vi "[Comment] Write.vi"(8 "error in (no error)":errorcluster, 11 "Graph Comment Config":T2[](array[typedef])) -> (0 "error out":errorcluster)   [LabVIEW 2019, in "Graph Tools.lvlib"]
uses:
  Graph Tools.lvlib
  [Comment] Config.ctl
  Selection VIs/controls/MarkerOptions.ctl
  <vilib>/Utility/miscctls.llb/LVPoint32TypeDef.ctl
  Selection VIs/controls/MarkerInfo.ctl
  Selection VIs/controls/markerType.ctl
panel:
  out "Coords":T1
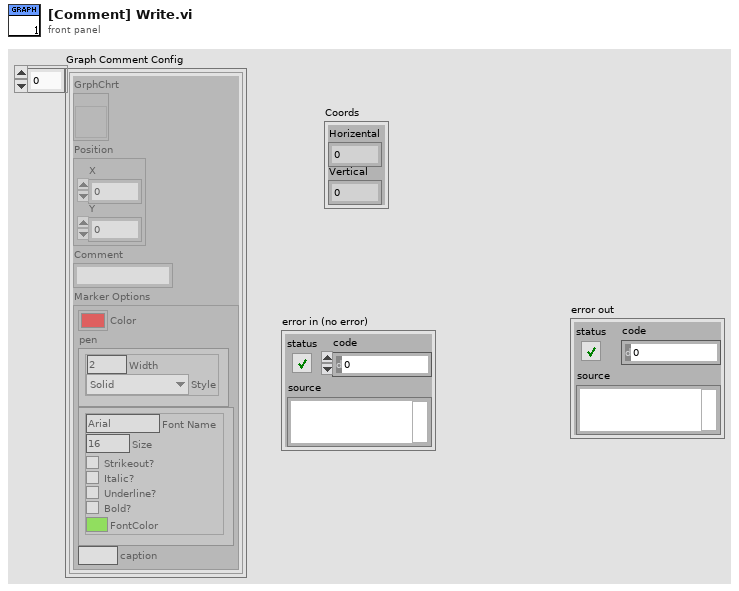
[diagram p1: front panel]
types:
  T1 = typedef "LVPoint32TypeDef.ctl" = cluster{"Horizental":i32, "Vertical":i32}
  T2 = typedef "Graph Tools.lvlib/[Comment] Config.ctl" = cluster{"GrphChrt":refnum<vi>, "Position":cluster{"X":dbl, "Y":dbl}, "Comment":string, "Marker Options":T3}
  T3 = typedef "MarkerOptions.ctl" = cluster{"Color":u32, "pen":cluster{"Width":u16, "Style":enum32{"Solid", "Dash", "Dot", "DashDot", "DashDotDot"}}, "font":cluster{"Font Name":string, "Size":i16, "Strikeout?":bool, "Italic?":bool, "Underline?":bool, "Outline?":bool, "Shadow?":bool, "Bold?":bool, "FontColor":u32}, "caption":string}
  T4 = typedef "MarkerInfo.ctl" = cluster{"Type":T5, "X":dbl, "Y":dbl, "X2":dbl, "Y2":dbl, "Text":string}
  T5 = typedef "markerType.ctl" = enum16{"point", "arrow", "horiz", "vert", "vert range", "horiz range", "box"}
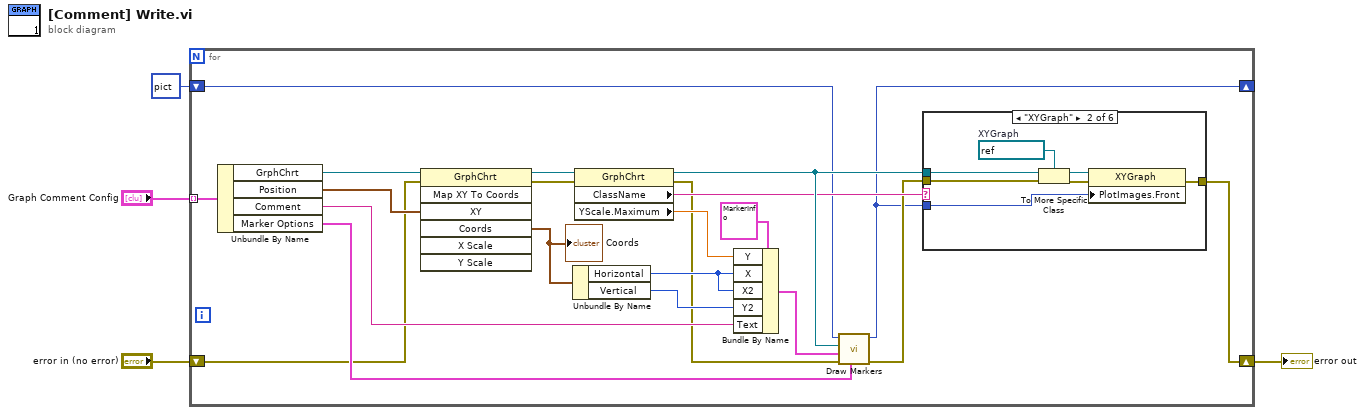
[diagram p0: block diagram]
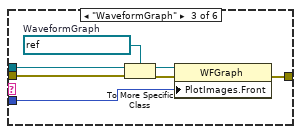
[diagram p3: hidden frame]
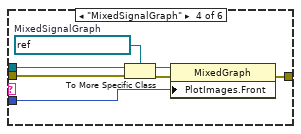
[diagram p4: hidden frame]
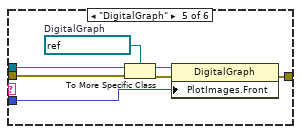
[diagram p5: hidden frame]
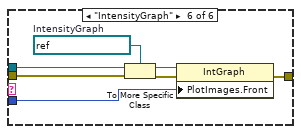
[diagram p6: hidden frame]
diagram:
  n1 = for {
    tunnel: "Graph Comment Config" -> [w13] mode=indexing
    shift-right: [w17] -> w2
    shift-left: "error in (no error)" -> [w5]
    shift-right: [w12] -> _
    shift-left: picture data[5B] ("Picture out") -> [w11]
    n2 = Unbundle By Name(w13) -> ("GrphChrt"=w10:refnum<vi>, "Position"=w9:cluster{"X":dbl, "Y":dbl}, "Comment"=w16:string, "Marker Options"=w15:T3)
    n3 = invoke class="GrphChrt" method="Map XY To Coords"(reference=w10, error in=w5, "XY"=w9) -> (reference out=w7:refnum<vi>, error out=w6:errorcluster, "Coords"=w8:T1)  [unwired: 4 in, 4 out]
    "Coords" <- w8
    n4 = Unbundle By Name(w8) -> ("Horizontal"=w24:i32, "Vertical"=w23:i32)
    n5 = property class="GrphChrt"(reference=w7, error in=w6) -> (reference out=w21:refnum<vi>, error out=w14:errorcluster, "ClassName"=w20:string, "YScale.Maximum"=w18:dbl)
    n6 = Bundle By Name(cluster=T4 {"Type"=enum."arrow", "X"=0.0, "Y"=0.0, "X2"=0.0, "Y2"=0.0, "Text"="Comment"} ("Marker"), "Y"=w18, "X"=w24, "X2"=w24, "Y2"=w23, "Text"=w16) -> (w22:T4)
    n7 = call "Draw Markers.vi"("Marker Options"=w15, "error in (no error)"=w14, "Marker"=w22, "GrphChrt Refnum"=w21, "picture"=w11) -> ("error out"=w19:errorcluster, "Picture out"=w12:picture)  [unwired: 5 in]
    n8 = case shown="\"XYGraph\"" w20 {
      tunnel: w21 -> [_ w33 w40 w47 w54 w61]
      tunnel: w19 -> [w26 w31 w38 w42 w49 w56]
      tunnel: w12 -> [_ w29 w34 w41 w48 w55]
      tunnel: [w26 w27 w36 w44 w51 w58] -> w17
      frame Default {
      }
      frame "XYGraph" {
        w32 = refnum<vi> refnum  # XYGraph
        n9 = To More Specific Class(target class=w32, reference=w33, error in=w31) -> (specific class reference=w30:refnum<vi>, error out=w28:errorcluster)
        n10 = property class="XYGraph"(reference=w30, error in=w28, "PlotImages.Front"=w29) -> (error out=w27:errorcluster)  [unwired: 1 out]
      }
      frame "WaveformGraph" {
        w39 = refnum<vi> refnum  # WaveformGraph
        n11 = To More Specific Class(target class=w39, reference=w40, error in=w38) -> (specific class reference=w37:refnum<vi>, error out=w35:errorcluster)
        n12 = property class="WFGraph"(reference=w37, error in=w35, "PlotImages.Front"=w34) -> (error out=w36:errorcluster)  [unwired: 1 out]
      }
      frame "MixedSignalGraph" {
        w46 = refnum<vi> refnum  # MixedSignalGraph
        n13 = To More Specific Class(target class=w46, reference=w47, error in=w42) -> (specific class reference=w45:refnum<vi>, error out=w43:errorcluster)
        n14 = property class="MixedGraph"(reference=w45, error in=w43, "PlotImages.Front"=w41) -> (error out=w44:errorcluster)  [unwired: 1 out]
      }
      frame "DigitalGraph" {
        w53 = refnum<vi> refnum  # DigitalGraph
        n15 = To More Specific Class(target class=w53, reference=w54, error in=w49) -> (specific class reference=w52:refnum<vi>, error out=w50:errorcluster)
        n16 = property class="DigitalGraph"(reference=w52, error in=w50, "PlotImages.Front"=w48) -> (error out=w51:errorcluster)  [unwired: 1 out]
      }
      frame "IntensityGraph" {
        w60 = refnum<vi> refnum  # IntensityGraph
        n17 = To More Specific Class(target class=w60, reference=w61, error in=w56) -> (specific class reference=w59:refnum<vi>, error out=w57:errorcluster)
        n18 = property class="IntGraph"(reference=w59, error in=w57, "PlotImages.Front"=w55) -> (error out=w58:errorcluster)  [unwired: 1 out]
      }
    }
  }
  "error out" <- w2
